vi "Test Enum Helpers.vi"() -> ()   [LabVIEW 2013, in "Table Manager.lvlib"]
uses:
  Table Manager.lvlib
  Column/Column Type.ctl
  Column/Column.lvclass
panel:
  out "Value 3":i32
  out "Value 2":string
  out "data":i32
  in  "specific class reference":refnum<vi>
  out "Column Type 2":T1
  out "Value":i32
  in  "Column Type":T1
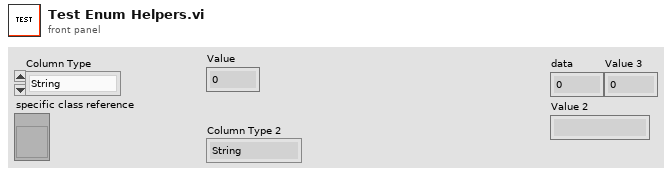
[diagram p1: front panel]
types:
  T1 = typedef "Table Manager.lvlib/Column.lvclass/Column Type.ctl" = enum16{"String", "Mapping", "Channel Name", "Tag", "Enum", "Data Type", "Numeric"}
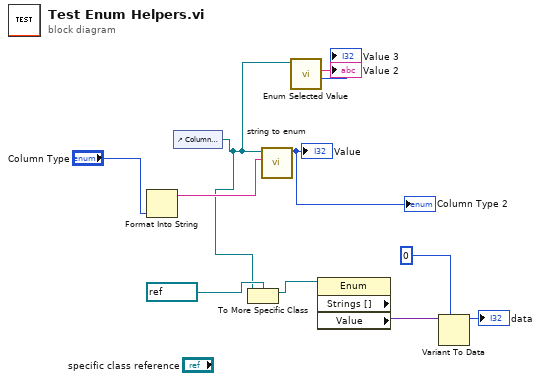
[diagram p0: block diagram]
diagram:
  n1 = Format Into String("Column Type") -> (resulting string=w10:string)  [unwired: 3 in, 1 out]
  n2 = control-ref of="Column Type"() -> (w3:refnum<vi>)
  n3 = To More Specific Class(target class=refnum<vi> refnum ("Enum"), reference=w3) -> (specific class reference=w7:refnum<vi>)  [unwired: 1 in, 1 out]
  n4 = call "string to enum.vi"("String"=w10, "Enum"=w3) -> ("Value"=→"Value" →"Column Type 2":i32)  [unwired: 8 in, 1 out]
  n5 = call "Enum Selected Value.vi"("Enum"=w3) -> (1:"Value"=→"Value 3":i32, 2:"Value"=→"Value 2":string)  [unwired: 8 in, 1 out]
  n6 = property class="Enum" props=["Strings []", "Value"](reference=w7) -> ("Value"=w6:variant)  [unwired: 1 in, 3 out]
  n7 = Variant To Data(type=0, Variant=w6) -> (data=→"data":i32)  [unwired: 1 in, 1 out]
